vi "InstConfigToSetupStr.vi"(8 "Setups":T1(array[cluster]), 11 "Configuration":T2 {"Select Mode:" items=["Custom", "Imaging", "300 All", "600 UV", "600 Blue", "600 Mid", "600 Red", "1200 m0", "1200 m1", "1200 m2", "1200 m3", "1200 m4", "1200 m5", "1200 m6", "1200 m7", "1200 RESOLVE", "400 m1", "400 m2", "930 m1", "930 m2", "930 m3", "930 m4", "930 m5", "930 m6", "400KL"]}) -> (3 "Command":string)   [LabVIEW 2015]
uses:
  GSP_ObsConfig.llb/configuration.ctl
  Users/Sherman/Desktop/BETA_GSCS/GUI/GSP_GUI_global.vi
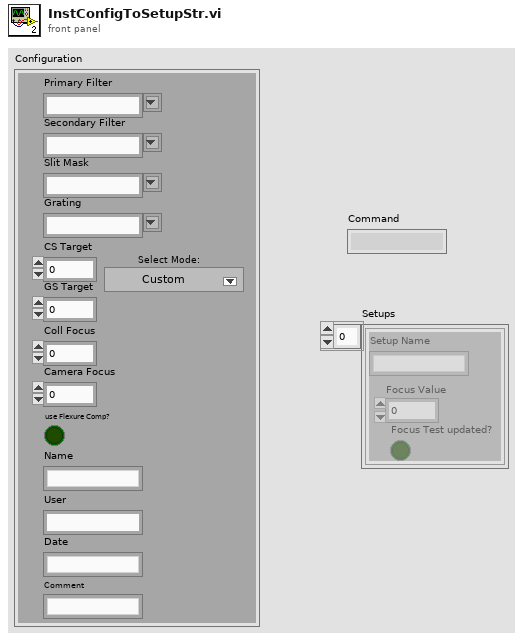
[diagram p1: front panel]
types:
  T1 = cluster{"Setup Name":string, "Focus Value":dbl, "Focus Test updated?":bool}[]
  T2 = typedef "configuration.ctl" = cluster{"Primary Filter":string, "Secondary Filter":string, "Slit Mask":string, "Grating":string, "CS Target":dbl, "GS Target":dbl, "Coll Focus":i32, "Camera Focus":i32, "Name":string, "User":string, "Date":string, "Comment":string, "use Flexure Comp?":bool, "Select Mode:":u16}
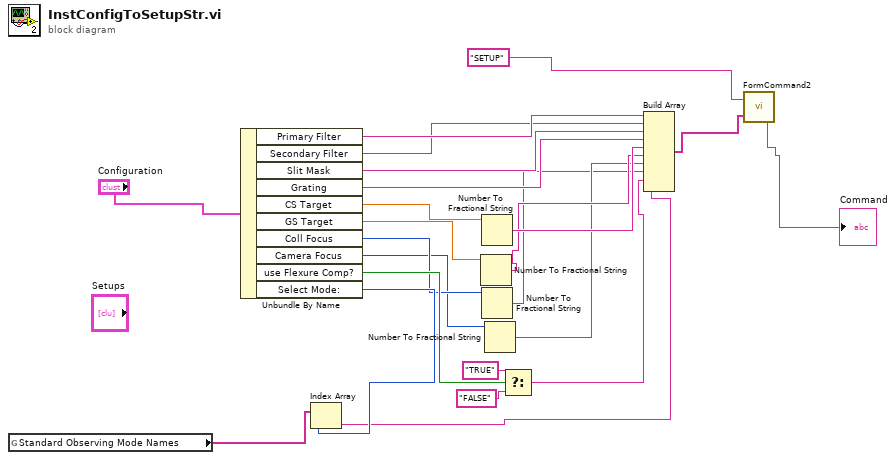
[diagram p0: block diagram]
diagram:
  n1 = global read "GSP_GUI_global.vi" "Standard Observing Mode Names"() -> (w20:string[])
  n2 = Unbundle By Name("Configuration") -> ("Primary Filter"=w13:string, "Secondary Filter"=w12:string, "Slit Mask"=w11:string, "Grating"=w10:string, "CS Target"=w22:dbl, "GS Target"=w21:dbl, "Coll Focus"=w9:i32, "Camera Focus"=w4:i32, "use Flexure Comp?"=w18:bool, "Select Mode:"=w19:u16)
  n3 = Index Array(array=w20, index=w19) -> (element=w14:string)
  n4 = Number To Fractional String(number=w21) -> (F-format string=w7:string)  [unwired: 3 in]
  n5 = Number To Fractional String(number=w22) -> (F-format string=w8:string)  [unwired: 3 in]
  n6 = Number To Fractional String(number=w9) -> (F-format string=w5:string)  [unwired: 3 in]
  n7 = Number To Fractional String(number=w4) -> (F-format string=w6:string)  [unwired: 3 in]
  n8 = Select(t="TRUE", s=w18, f="FALSE") -> (s? t:f=w15:string)
  n9 = Build Array(w13, w12, w11, w10, w8, w7, w6, w5, w15, w14) -> (w2:string[])
  n10 = call "FormCommand2.vi"("Parameters"=w2, "Command"="SETUP") -> ("Command string"=→"Command":string)
